vi "get_as_float.vi"(8 "error in (no error)":errorcluster, 11 "Image in":refnum<class "Image.lvclass">) -> (0 "error out":errorcluster, 2 "data":sgl[][](array[numeric]), 3 "Image out":refnum<class "Image.lvclass">)   [LabVIEW 2017, in "Image.lvclass"]
uses:
  Image.lvclass
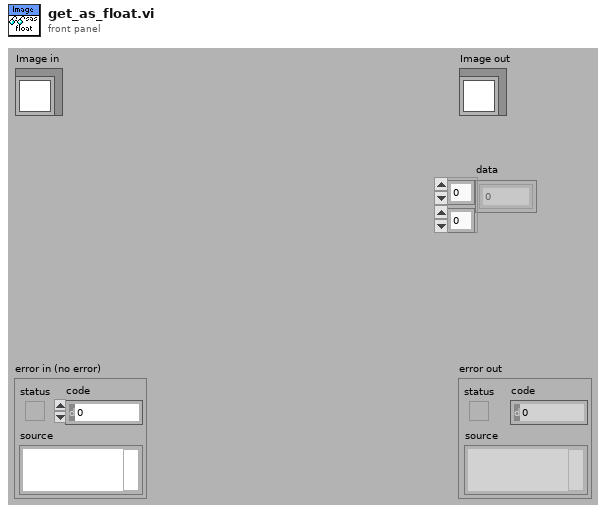
[diagram p1: front panel]
types:
  T1 = typedef "Image Type" = u32
  T2 = typedef "Color (U64)" = cluster{"Plane 3 (Blue)":u16, "Plane 2 (Green)":u16, "Plane 1 (Red)":u16, "Plane 4 (alpha)":u16}
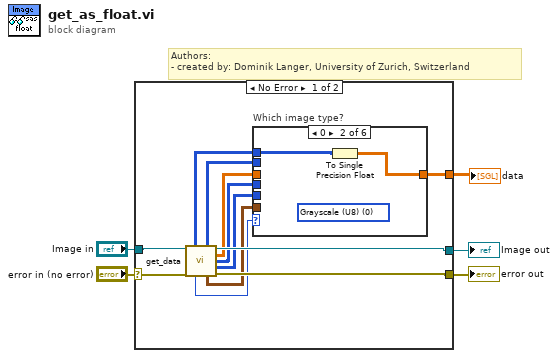
[diagram p0: block diagram]
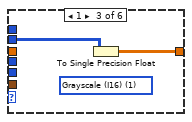
[diagram p3: hidden frame]
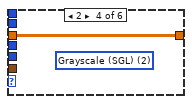
[diagram p4: hidden frame]
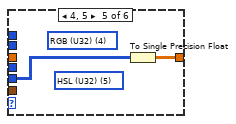
[diagram p5: hidden frame]
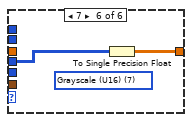
[diagram p6: hidden frame]
diagram:
  # "Authors: \n- created by: Dominik Langer, University of Zurich, Switzerland"
  n1 = case shown="No Error" "error in (no error)" {
    selector: "error in (no error)" -> [w13 w28]
    tunnel: [w17 w28] -> w4
    tunnel: [w14 w27] -> w2
    tunnel: "Image in" -> [w12 w27]
    tunnel: [w9 _] -> w1
    frame No Error {
      n2 = call-dynamic "get_data.vi"("Image in"=w12, "error in (no error)"=w13) -> ("Image Pixels (U8)"=w16:u8[][], "Image Pixels (I16)"=w15:i16[][], "Image out"=w14:refnum<class "Image.lvclass">, "Image Pixels (Float)"=w10:sgl[][], "Image Pixels (U16)"=w8:u16[][], "Image Pixels (U32)"=w7:u32[][], "Image Type"=w11:T1, "Image Pixels (U64)"=w6:T2[][], "error out"=w17:errorcluster)  [unwired: 5 in]
      n3 = case "Which image type?" shown="0" w11 {
        tunnel: w16 -> [_ w19 _ _ _ _]
        tunnel: w15 -> [_ _ w20 _ _ _]
        tunnel: w10 -> [_ _ _ w22 _ _]
        tunnel: [_ w18 w21 w22 w23 w26] -> w9
        tunnel: w8 -> [_ _ _ _ _ w25]
        tunnel: w7 -> [_ _ _ _ w24 _]
        tunnel: w6 -> [_ _ _ _ _ _]
        frame Default {
        }
        frame 0 {
          (unwired) T1 0 items=["Grayscale (U8)", "Grayscale (I16)", "Grayscale (SGL)", "Complex (CSG)", "RGB (U32)", "HSL (U32)", "RGB (U64)", "Grayscale (U16)"] ("target image type")
          n4 = To Single Precision Float(number=w19) -> (single precision float=w18:sgl[][])
        }
        frame 1 {
          (unwired) T1 1 items=["Grayscale (U8)", "Grayscale (I16)", "Grayscale (SGL)", "Complex (CSG)", "RGB (U32)", "HSL (U32)", "RGB (U64)", "Grayscale (U16)"] ("target image type")
          n5 = To Single Precision Float(number=w20) -> (single precision float=w21:sgl[][])
        }
        frame 2 {
          (unwired) T1 2 items=["Grayscale (U8)", "Grayscale (I16)", "Grayscale (SGL)", "Complex (CSG)", "RGB (U32)", "HSL (U32)", "RGB (U64)", "Grayscale (U16)"] ("target image type")
        }
        frame 4, 5 {
          (unwired) T1 4 items=["Grayscale (U8)", "Grayscale (I16)", "Grayscale (SGL)", "Complex (CSG)", "RGB (U32)", "HSL (U32)", "RGB (U64)", "Grayscale (U16)"] ("target image type")
          (unwired) T1 5 items=["Grayscale (U8)", "Grayscale (I16)", "Grayscale (SGL)", "Complex (CSG)", "RGB (U32)", "HSL (U32)", "RGB (U64)", "Grayscale (U16)"] ("target image type")
          n6 = To Single Precision Float(number=w24) -> (single precision float=w23:sgl[][])
        }
        frame 7 {
          (unwired) T1 7 items=["Grayscale (U8)", "Grayscale (I16)", "Grayscale (SGL)", "Complex (CSG)", "RGB (U32)", "HSL (U32)", "RGB (U64)", "Grayscale (U16)"] ("target image type")
          n7 = To Single Precision Float(number=w25) -> (single precision float=w26:sgl[][])
        }
      }
    }
    frame Error {
    }
  }
  "error out" <- w4
  "Image out" <- w2
  "data" <- w1
